vi "Strip Path Extension String.vi"(0 "path":string) -> (1 "root":string, 2 "extension":string)   [LabVIEW 2012, in "Path Function.lvlib"]
uses:
  Path Function.lvlib
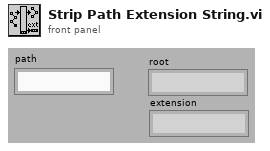
[diagram p1: front panel]
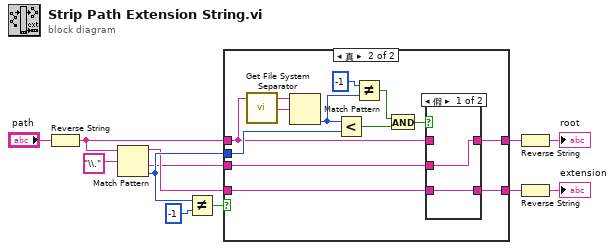
[diagram p0: block diagram]
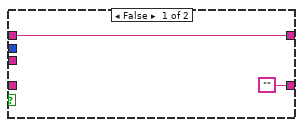
[diagram p2: hidden frame]
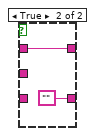
[diagram p3: hidden frame]
diagram:
  n1 = Reverse String(1:"path") -> (0:w1:string)
  n2 = Match Pattern(string=w1, regular expression="\\.") -> (before substring=w7:string, after substring=w6:string, offset past match=w8:i32)  [unwired: 1 in, 1 out]
  n3 = Not Equal?(x=w8, y=-1) -> (x != y?=w10:bool)
  n4 = case "Has Period?" shown="真" w10 {
    tunnel: w1 -> [w14 w19]
    tunnel: ["" w17] -> w3
    tunnel: [w14 w18] -> w5
    tunnel: w8 -> [_ w23]
    tunnel: w7 -> [_ w16]
    tunnel: w6 -> [_ w15]
    frame False {
    }
    frame True {
      n5 = call <vilib>:"Get File System Separator.vi"() -> ("Path Separator"=w26:string)
      n6 = Match Pattern(string=w19, regular expression=w26) -> (offset past match=w24:i32)  [unwired: 1 in, 3 out]
      n7 = Less?(x=w24, y=w23) -> (x < y?=w21:bool)
      n8 = Not Equal?(x=-1 ("y"), y=w24) -> (x != y?=w22:bool)
      n9 = And(x=w22, y=w21) -> (x .and. y?=w20:bool)
      n10 = case "Path Separator\nbefore Period?" shown="假" w20 {
        tunnel: w19 -> [_ w30]
        tunnel: [w28 w30] -> w18
        tunnel: [w27 ""] -> w17
        tunnel: w16 -> [w27 _]
        tunnel: w15 -> [w28 _]
        frame False {
        }
        frame True {
        }
      }
    }
  }
  n11 = Reverse String(1:w5) -> (0:→"root":string)
  n12 = Reverse String(1:w3) -> (0:→"extension":string)
